vi "Get Boolean.vi"(8 "error in (no error)":errorcluster, 10 "Name":string, 11 "json class in":refnum<class "json class.lvclass">) -> (0 "error out":errorcluster, 2 "Boolean":bool, 3 "json class out":refnum<class "json class.lvclass">)   [LabVIEW 2025, in "Config Library.lvlib" / "json class.lvclass"]
uses:
  json class.lvclass
  json class.lvclass/json class.ctl
  <vilib>/addons/JSON API/JSON Scalar/JSON Scalar.lvclass
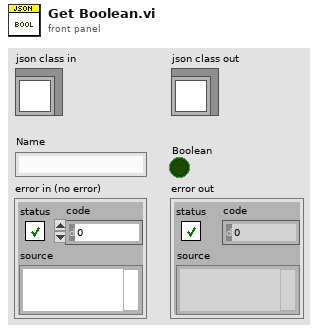
[diagram p1: front panel]
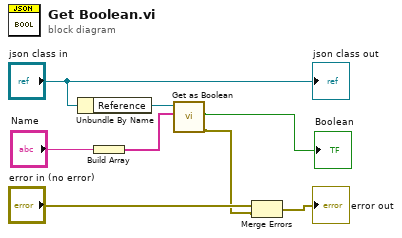
[diagram p0: block diagram]
diagram:
  n1 = Unbundle By Name("json class in") -> ("Reference"=w4:refnum<class "JSON Value.lvclass">)
  n2 = Build Array("Name") -> (w3:string[])
  n3 = call <vilib>:"Get as Boolean.vi"("Name Array"=w3, "JSON Value in"=w4) -> ("error out"=w2:errorcluster, "Boolean"=→"Boolean":bool)  [unwired: 7 in, 1 out]
  n4 = Merge Errors("error in (no error)", w2) -> (→"error out":errorcluster)
  "json class out" <- "json class in"
